vi "Calculate_Cost_F()-5.vi"(4 "[IN] Dot matrix with statuses \nfor potentially moving dots":i16[][](array[numeric]), 6 "[IN] Potentially\nMoving (X,Y)":dbl[][](array[numeric]), 7 "[IN] Max angle":dbl, 8 "error IN":errorcluster, 9 "[IN] Areas particles\nPrimary Detected":dbl[][](array[numeric]), 10 "[IN] Primary \n(X,Y) Detected":dbl[][](array[numeric]), 11 "[IN] Subtracks in Row":T1(array[cluster])) -> (0 "error OUT":errorcluster, 3 "[OUT] Cost function":i8[](array[numeric]))   [LabVIEW 2013]
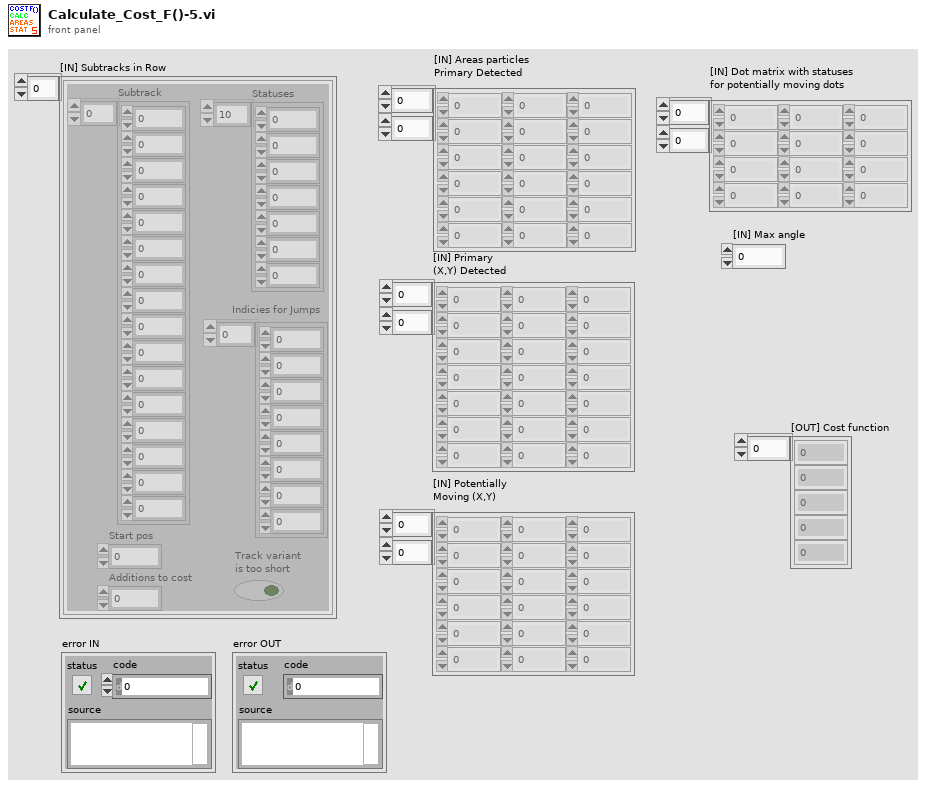
[diagram p1: front panel]
types:
  T1 = cluster{"Subtrack":dbl[], "Statuses":i16[], "Start pos":i32, "Additions to cost":i8, "Track variant \nis too short":bool, "Indicies for Jumps":i32[]}[]
  T2 = cluster{"Subtrack":dbl[], "Statuses":i16[], "Start pos":i32, "Additions to cost":i8, "Track variant \nis too short":bool, "Indicies for Jumps":i32[]}
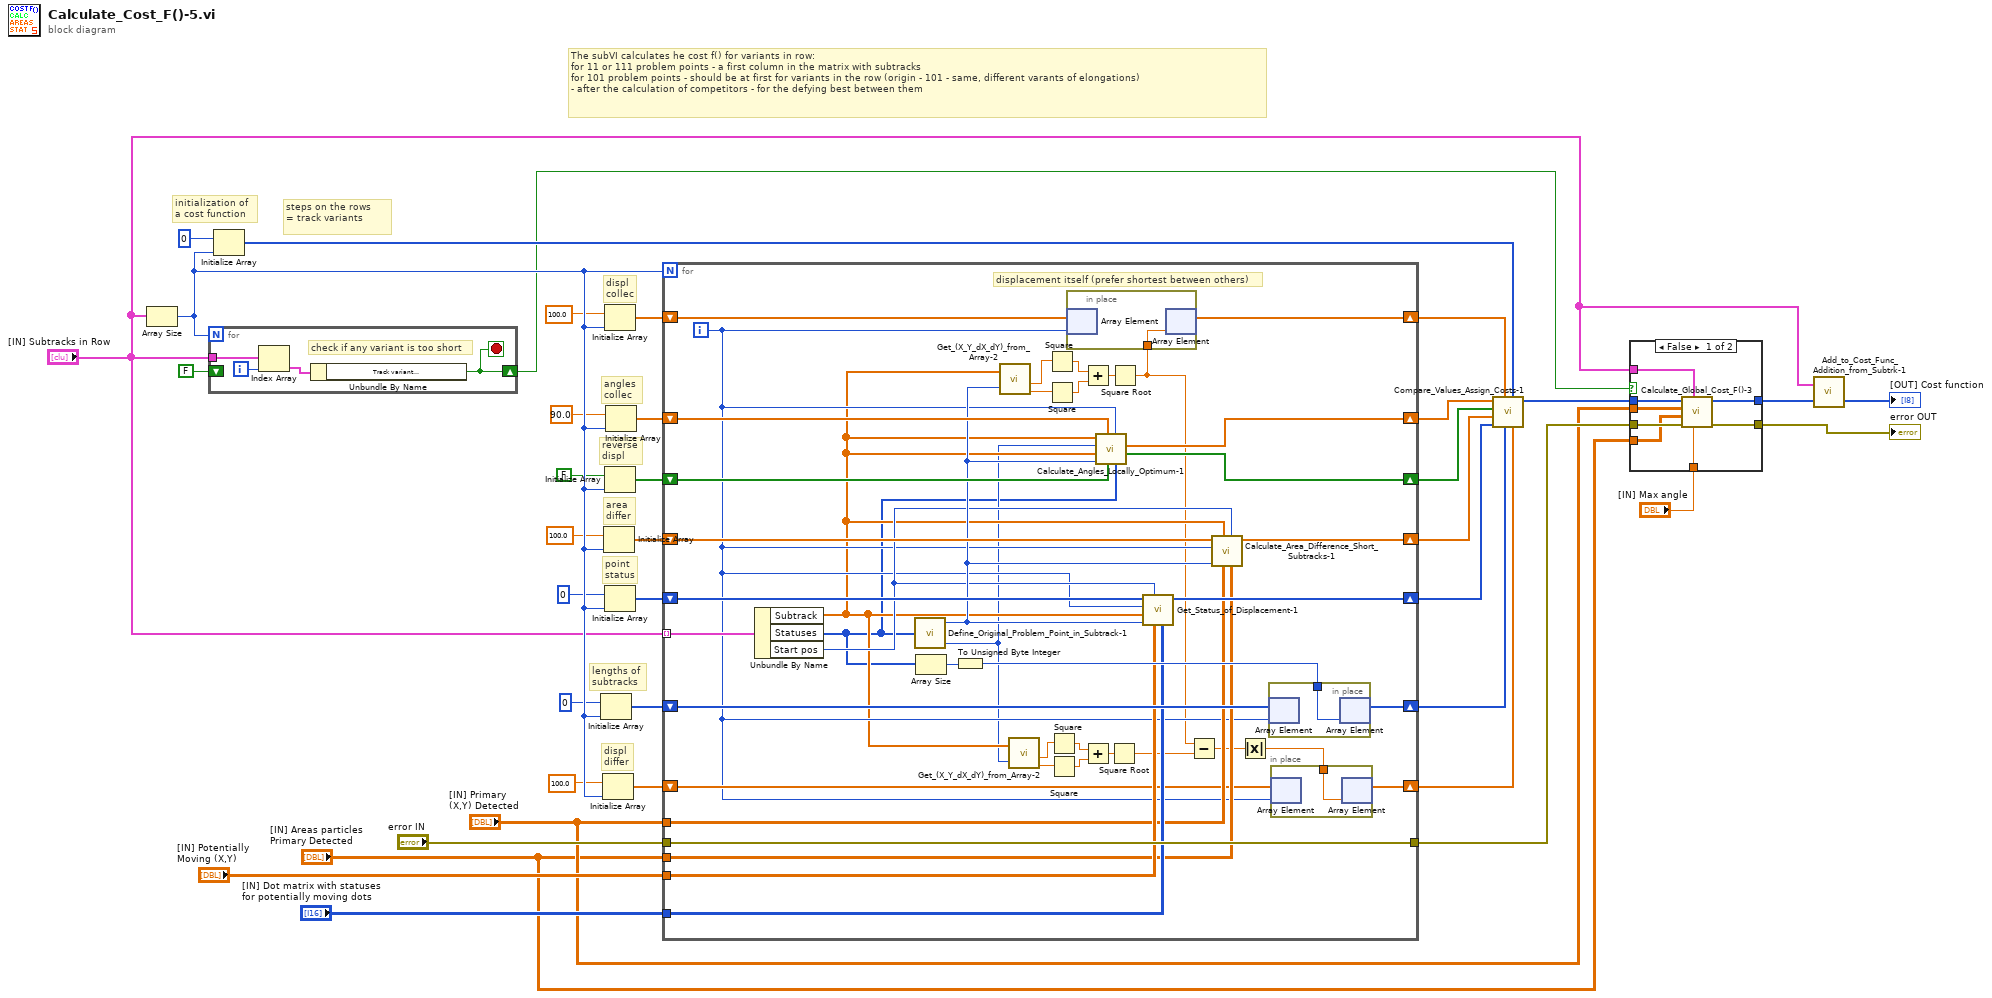
[diagram p0: block diagram]
diagram:
  # "displ \ndiffer"
  # "lengths of\nsubtracks"
  # "point\nstatus"
  # "area \ndiffer"
  # "reverse \ndispl"
  # "angles \ncollec"
  # "displ \ncollec"
  # "The subVI calculates he cost f() for variants in row:\nfor 11 or 111 problem points - a first column in the matrix with subtracks\nfor 101 problem points - should be at first for variants in the row (origin - 101 - same, different varants of elongations)\n- after the calculation of competitors - for the defying best between them"
  # "initialization of \na cost function"
  # "steps on the rows\n= track variants"
  n1 = Array Size(array="[IN] Subtracks in Row") -> (size(s)=w32:i32)
  n2 = for {
    N: w32 -> [_]
    shift-right: [w39] -> w8
    shift-left: FALSE -> [_]
    tunnel: "[IN] Subtracks in Row" -> [w42]
    i -> [w41]
    stop <- w39 stop-if-true
    # "check if any variant is too short"
    n3 = Index Array(array=w42, index=w41) -> (element=w40:T2)
    n4 = Unbundle By Name(w40) -> ("Track variant \nis too short"=w39:bool)
  }
  n5 = Initialize Array(i8 0, w32) -> (w33:i8[])
  n6 = Initialize Array(u8 0, w32) -> (w20:u8[])
  n7 = Initialize Array(100.0, w32) -> (w18:dbl[])
  n8 = Initialize Array(100.0, w32) -> (w24:dbl[])
  n9 = Initialize Array(100.0, w32) -> (w30:dbl[])
  n10 = Initialize Array(FALSE, w32) -> (w26:bool[])
  n11 = Initialize Array(i16 0, w32) -> (w22:i16[])
  n12 = Initialize Array(90.0, w32) -> (w28:dbl[])
  n13 = for {
    N: w32 -> [_]
    shift-right: [w76] -> w16
    shift-left: w30 -> [w82]
    shift-right: [w69] -> w17
    shift-left: w28 -> [w71]
    shift-right: [w68] -> w15
    shift-left: w26 -> [w70]
    tunnel: "[IN] Primary \n(X,Y) Detected" -> [w61]
    tunnel: "[IN] Areas particles\nPrimary Detected" -> [w60]
    shift-right: [w58] -> w14
    shift-left: w24 -> [w63]
    tunnel: "[IN] Potentially\nMoving (X,Y)" -> [w66]
    tunnel: "[IN] Dot matrix with statuses \nfor potentially moving dots" -> [w65]
    shift-right: [w64] -> w13
    shift-left: w22 -> [w67]
    tunnel: "error IN" -> [w84]
    tunnel: [w84] -> w9
    shift-right: [w72] -> w12
    shift-left: w20 -> [w75]
    tunnel: "[IN] Subtracks in Row" -> [w83] mode=indexing
    shift-right: [w53] -> w11
    shift-left: w18 -> [w57]
    i -> [w56]
    # "displacement itself (prefer shortest between others)"
    n14 = Unbundle By Name(w83) -> ("Subtrack"=w55:dbl[], "Statuses"=w43:i16[], "Start pos"=w59:i32)
    n15 = call "Define_Original_Problem_Point_in_Subtrack-1.vi"("[IN] Statuses"=w43) -> ("[OUT] Index of Displace\nment Before or After"=w54:i32, "[OUT] Index of Problem Point\nin Subtrack (Original)"=w62:i32)  [unwired: 3 in]
    n16 = Array Size(array=w43) -> (size(s)=w74:i32)
    n17 = To Unsigned Byte Integer(number=w74) -> (unsigned 8bit integer=w73:u8)
    n18 = call "Get_(X_Y_dX_dY)_from_Array-2.vi"("(X,Y,dX,dY)"=w55, "Index of Displacement"=w62) -> ("dX"=w80:dbl, "dY"=w81:dbl)  [unwired: 2 out]
    n19 = call "Get_(X_Y_dX_dY)_from_Array-2.vi"("(X,Y,dX,dY)"=w55, "Index of Displacement"=w54) -> ("dX"=w49:dbl, "dY"=w48:dbl)  [unwired: 2 out]
    n20 = Square(x=w80) -> (x^2=w77:dbl)
    n21 = Square(x=w81) -> (x^2=w78:dbl)
    n22 = Square(x=w49) -> (x^2=w50:dbl)
    n23 = Square(x=w48) -> (x^2=w51:dbl)
    n24 = Add(x=w77, y=w78) -> (x+y=w79:dbl)
    n25 = Add(x=w50, y=w51) -> (x+y=w52:dbl)
    n26 = call "Calculate_Angles_Locally_Optimum-1.vi"("Statuses"=w43, "[IN] Index of subtrack"=w56, "[IN] Reverse Displ or Not"=w70, "[IN] Array with Angles \nBetween Displacement"=w71, "[IN] Index of Cur\nrent Displacement"=w62, "[IN] Track with \nCurrent Point"=w55, "[IN] Index of Previ\nous Displacement"=w54, "[IN] Track with \nPrevious Point"=w55) -> ("[OUT] Reverse displacement or not"=w68:bool[], "[OUT] Angles betwe\nen two displacements"=w69:dbl[])  [unwired: 2 in]
    n27 = Square Root(x=w52) -> (sqrt(x)=w46:dbl)
    n28 = Square Root(x=w79) -> (sqrt(x)=w47:dbl)
    n29 = in-place {
      in-place-border: w47 -> [w87]
      n30 = in-place-array #1(w82, w56) -> ()  [unwired: 1 out]
      n31 = in-place-array #1(w87) -> (w76:dbl[])  [unwired: 1 out]
    }
    n32 = call "Get_Status_of_Displacement-1.vi"("[IN] Dot matrix with statuses\nfor potentially moving dots"=w65, "[IN] Potentially\nMoving (X,Y)"=w66, "[IN] Start pos"=w59, "[IN] Index of Problem\nPoint in Subtrack"=w62, "[IN] Subtrack"=w55, "[IN] Index of\n subtrack"=w56, "[IN] Displace-\nment Statuses"=w67) -> ("[OUT] Displace\nment Statuses"=w64:i16[])  [unwired: 4 in]
    n33 = Subtract(x=w47, y=w46) -> (x-y=w45:dbl)
    n34 = call "Calculate_Area_Difference_Short_Subtracks-1.vi"("[IN] Areas particles\nPrimary Detected"=w60, "[IN] Start pos"=w59, "[IN] Primary \n(X,Y) Detected"=w61, "[IN] Subtrack"=w55, "[IN] Index of \"11\" Dis-\nplacement in Subtrack"=w62, "[IN] Index of\n subtrack"=w56, "[IN] Areas \ndifference"=w63) -> ("[OUT] Areas \ndifference"=w58:dbl[])  [unwired: 4 in]
    n35 = Absolute Value(x=w45) -> (abs(x)=w44:dbl)
    n36 = in-place {
      in-place-border: w73 -> [w86]
      n37 = in-place-array #2(w75, w56) -> ()  [unwired: 1 out]
      n38 = in-place-array #2(w86) -> (w72:u8[])  [unwired: 1 out]
    }
    n39 = in-place {
      in-place-border: w44 -> [w85]
      n40 = in-place-array #3(w57, w56) -> ()  [unwired: 1 out]
      n41 = in-place-array #3(w85) -> (w53:dbl[])  [unwired: 1 out]
    }
  }
  n42 = call "Compare_Values_Assign_Costs-1.vi"("[IN] Array of displa\ncement differences"=w11, "[IN] Cost function"=w33, "[IN] Track Length"=w12, "[IN] Array of displacements"=w16, "[IN] Statuses of points"=w13, "[IN] Areas \ndifferences"=w14, "[IN] Reverse or not"=w15, "[IN] Angles betwe\nen displacements"=w17) -> ("[OUT] Cost function"=w10:i8[])  [unwired: 3 in]
  n43 = case shown="False" w8 {
    tunnel: w10 -> [w94 w97]
    tunnel: w9 -> [w92 w96]
    tunnel: "[IN] Max angle" -> [w95 _]
    tunnel: [w93 w97] -> w3
    tunnel: [w91 w96] -> w4
    tunnel: "[IN] Subtracks in Row" -> [w90 _]
    tunnel: "[IN] Primary \n(X,Y) Detected" -> [w89 _]
    tunnel: "[IN] Areas particles\nPrimary Detected" -> [w88 _]
    frame False {
      n44 = call "Calculate_Global_Cost_F()-3.vi"("[IN] Max angle"=w95, "[IN] Subtracks in Row"=w90, "error IN"=w92, "[IN] Areas particles\nPrimary Detected"=w88, "[IN] Primary \n(X,Y) Detected"=w89, "[IN] Cost function"=w94) -> ("error OUT"=w91:errorcluster, "[OUT] Cost function"=w93:i8[])  [unwired: 4 in]
    }
    frame True {
    }
  }
  "error OUT" <- w4
  n45 = call "Add_to_Cost_Func_Addition_from_Subtrk-1.vi"("[IN] Cost function"=w3, "[IN] Subtracks in Row"="[IN] Subtracks in Row") -> ("[OUT] Cost function"=→"[OUT] Cost function":i8[])  [unwired: 1 in]
